vi "IR open.vi"(8 "error in (no error)":errorcluster, 10 "IR pin":T1(ring), 11 "IR sensor in":refnum<class "IR sensor.lvclass">) -> (0 "error out":errorcluster, 3 "IR sensor out":refnum<class "IR sensor.lvclass">)   [LabVIEW 2019, in "my FPGA lib.lvlib" / "IR sensor.lvclass"]
uses:
  IR sensor.lvclass
  IR sensor.lvclass/IR sensor.ctl
  my FPGA lib.lvlib
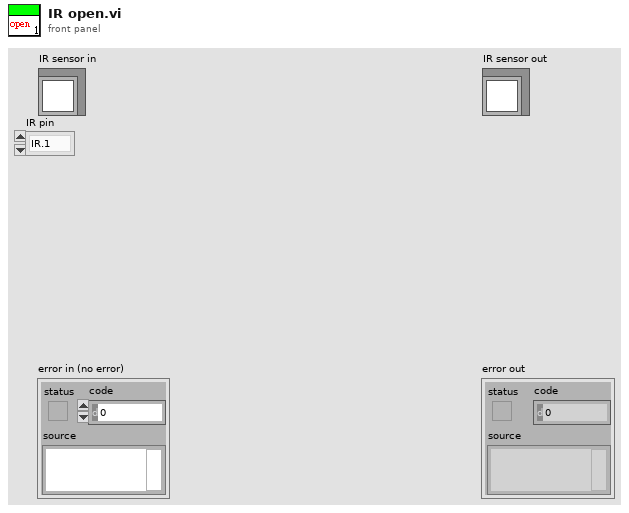
[diagram p1: front panel]
types:
  T1 = enum16{"IR.1", "IR.2", "IR.3", "IR.4", "IR.5", "IR.6", "IR.7", "IR.8"}
  T2 = typedef "my FPGA lib.lvlib/FPPGA.ctl" = refnum<k20>
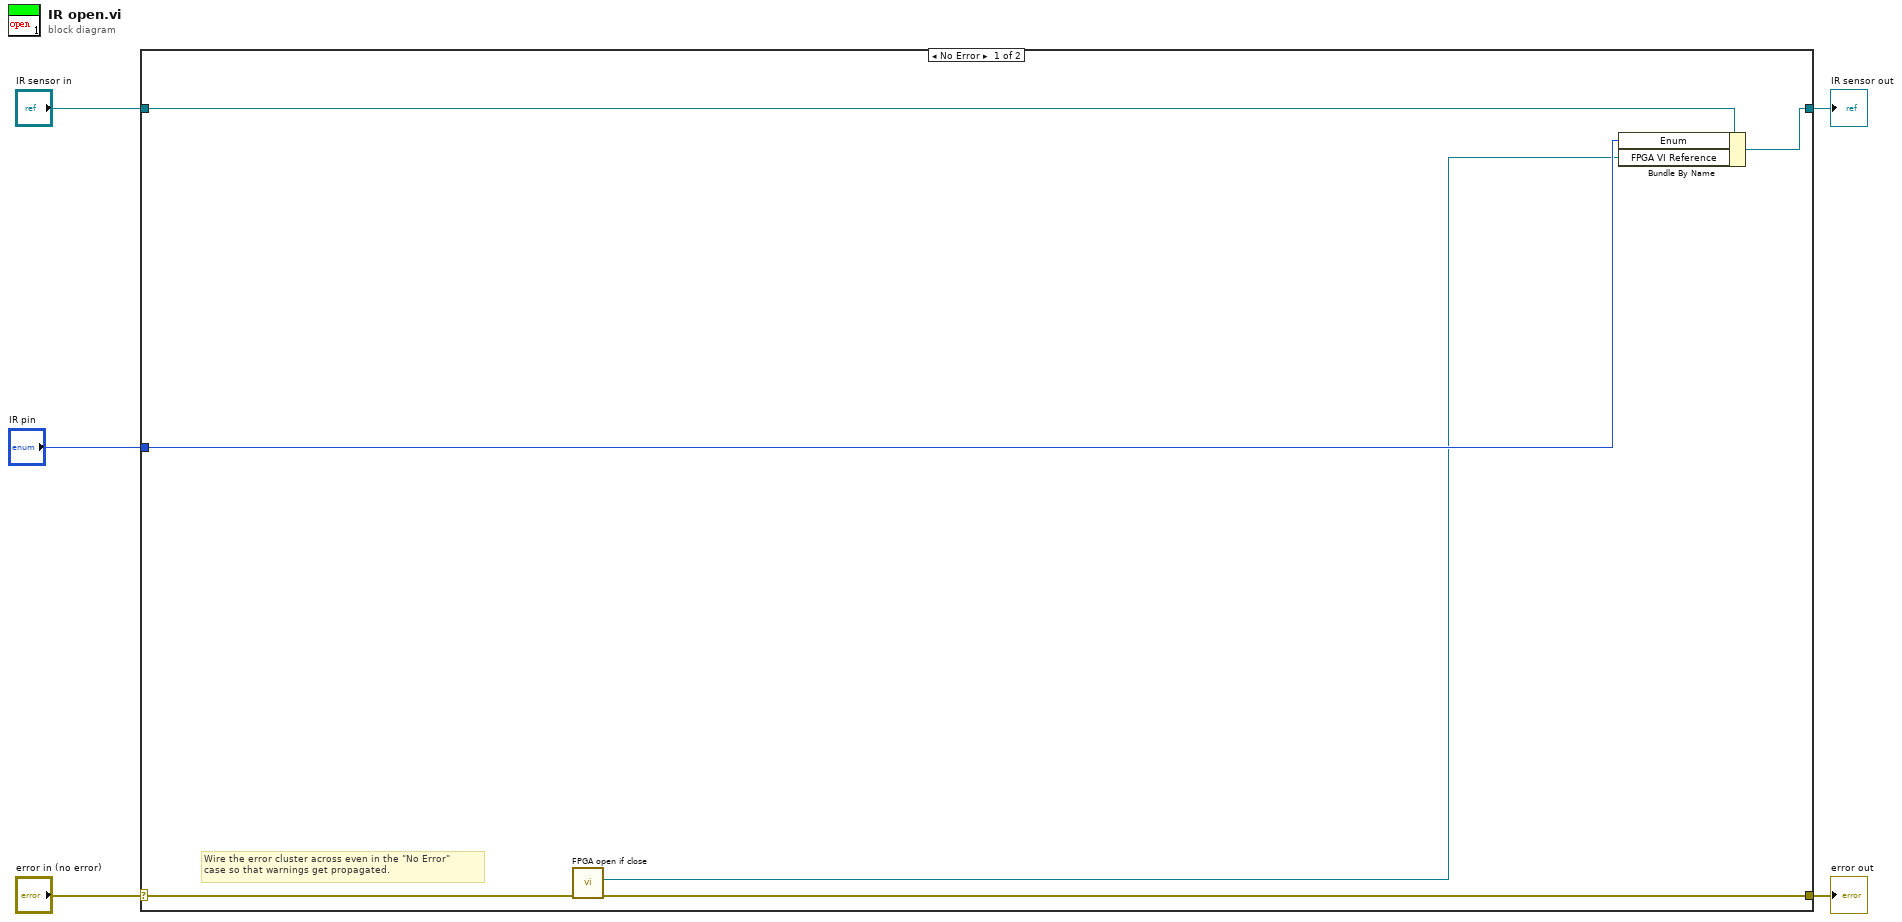
[diagram p0: block diagram]
diagram:
  n1 = case shown="No Error" "error in (no error)" {
    selector: "error in (no error)" -> [w8 w13]
    tunnel: [w7 w13] -> w4
    tunnel: [w10 w12] -> w2
    tunnel: "IR sensor in" -> [w11 w12]
    tunnel: "IR pin" -> [w9 _]
    frame No Error {
      # "Wire the error cluster across even in the \"No Error\"\ncase so that warnings get propagated."
      n2 = call "FPGA open if close.vi"("error in"=w8) -> ("error out"=w7:errorcluster, "FPGA VI Reference Out"=w6:T2)  [unwired: 9 in]
      n3 = Bundle By Name(cluster=w11, "Enum"=w9, "FPGA VI Reference"=w6) -> (w10:refnum<class "IR sensor.lvclass">)
    }
    frame Error {
    }
  }
  "error out" <- w4
  "IR sensor out" <- w2
